vi "Sensor Setting.vi"(8 "error in":errorcluster) -> (0 "error  out":errorcluster)   [LabVIEW 2015]
uses:
  Control Button/Save.ctl
  Control Button/Exit.ctl
  <vilib>/addons/database/Connection.llb/DB Tools Open Connec (String).vi
  Galobal variable_TI.vi
  <vilib>/addons/database/_DB Variant To Data/Database Variant To Data.xnode
  <vilib>/addons/database/NI_Database_API.lvlib
panel:
  out "error out":errorcluster
  in  "Model":string(combo)
  in  "Setting Data":T1
  in  "String":string
  in  "Cluster 3":T1
  out "Model":string
  in  "Exit":T2
  in  "Save":T3
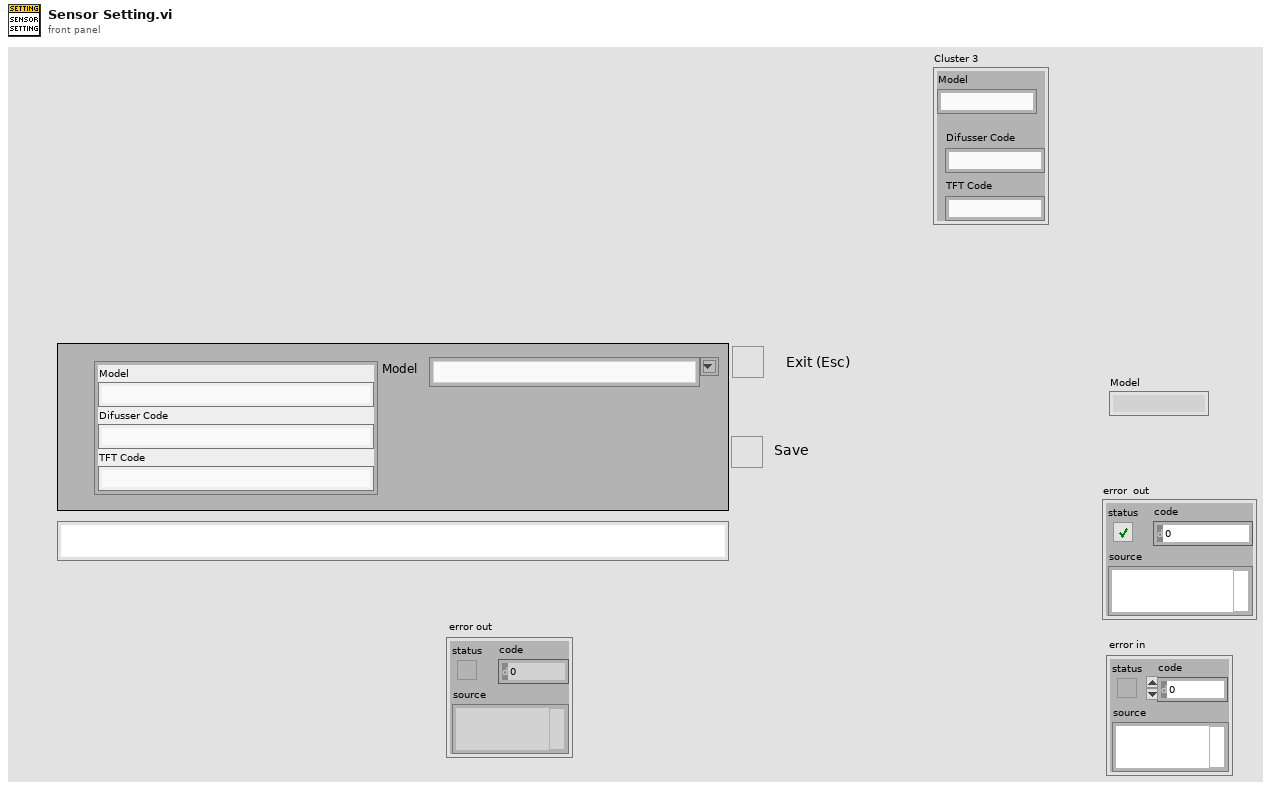
[diagram p1: front panel]
types:
  T1 = cluster{"Model":string, "Difusser Code":string, "TFT Code ":string}
  T2 = typedef "Exit.ctl" = bool
  T3 = typedef "Save.ctl" = bool
  T4 = typedef "NI_Database_API.lvlib/Conn ObjectReference.ctl" = refnum<k1>
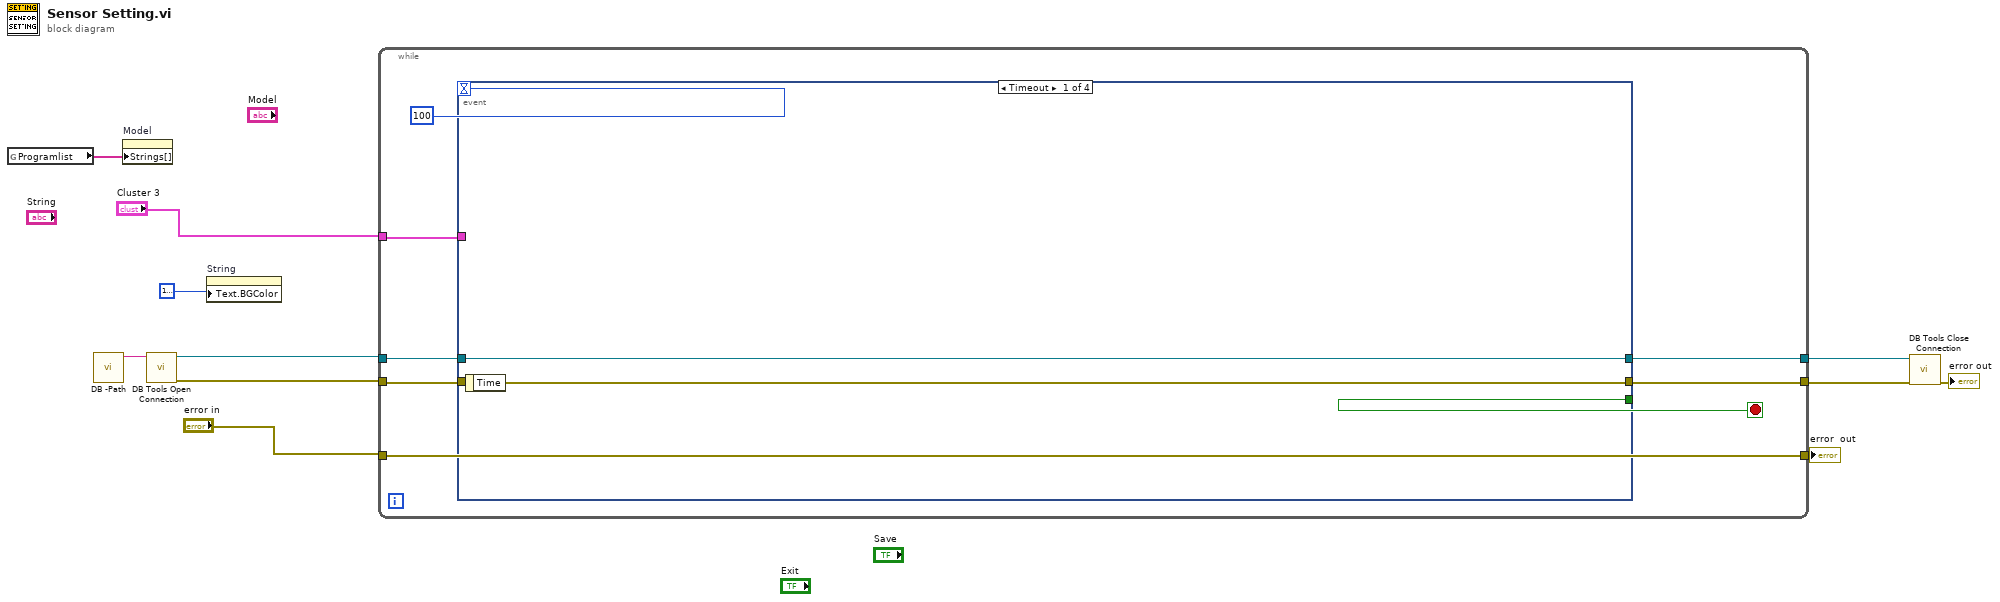
[diagram p0: block diagram]
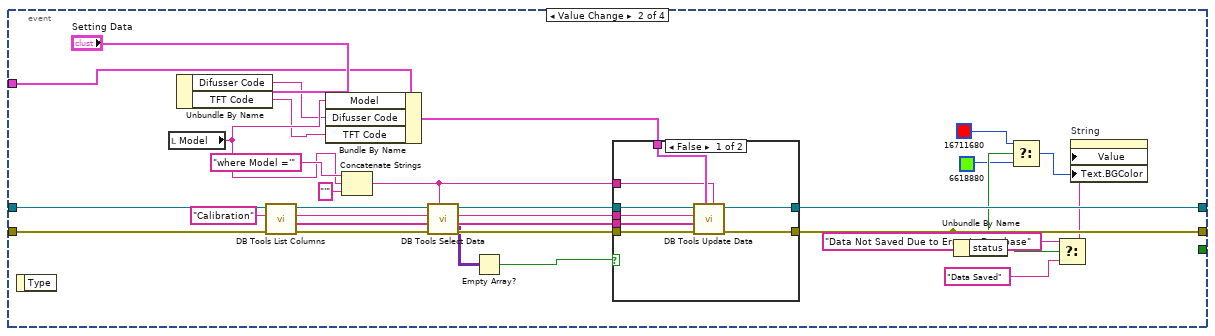
[diagram p2: hidden frame]
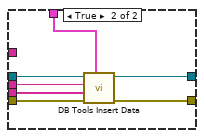
[diagram p3: hidden frame]
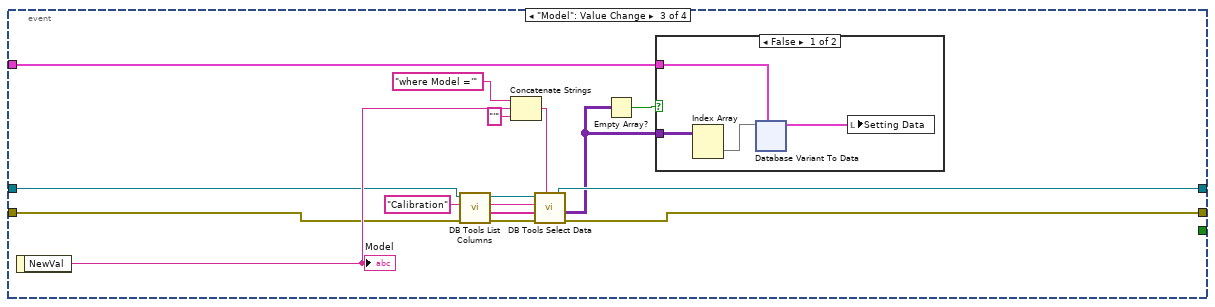
[diagram p4: hidden frame]
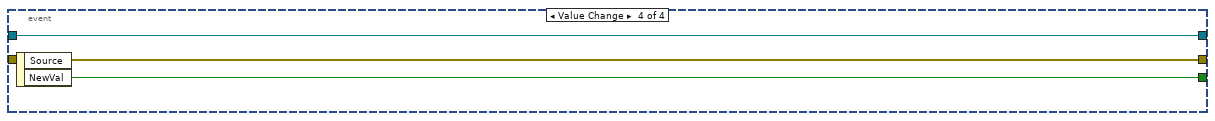
[diagram p6: hidden frame]
diagram:
  n1 = global read "Galobal variable_TI.vi" "Programlist"() -> (w6:string[])
  n2 = call "DB -Path.vi"() -> ("String"=w11:string)  [unwired: 11 in]
  n3 = property on="Model" class="CmbBox"("Strings[]"=w6) -> ()  [unwired: 2 in, 2 out]
  n4 = call-poly <vilib>:"DB Tools Open Connection.vi"("connection information"=w11) -> ("error out"=w9:errorcluster, "connection reference"=w10:T4)  [unwired: 7 in]
  n5 = property on="String" class="Str"("Text.BGColor"=u32 16777226 ("Color Box")) -> ()  [unwired: 2 in, 2 out]
  n6 = while {
    tunnel: w10 -> [w18]
    tunnel: w9 -> [w17]
    tunnel: [w16] -> w8
    tunnel: [w15] -> w7
    tunnel: "error in" -> [w13]
    tunnel: [w13] -> w4
    tunnel: "Cluster 3" -> [w12]
    stop <- w14 stop-if-true
    n7 = event shown="[0] Timeout" {
      selector: _ -> [_ _ _ _]
      dyn-events: _ -> [_ _ _ _]
      timeout: 100 -> [_ _ _ _]
      tunnel: w18 -> [w21 w49 w71 w182]
      tunnel: w17 -> [w20 w48 w70 w183]
      tunnel: [w21 w47 w69 w182] -> w16
      tunnel: [w20 w38 w68 w183] -> w15
      tunnel: [_ _ _ w181] -> w14
      tunnel: w12 -> [_ w41 w67 _]
      event Timeout {
        n8 = event-data() -> ()  [unwired: 1 in, 1 out]
      }
      event Value Change {
        w25 = "Calibration" ("table")
        n9 = event-data() -> ()  [unwired: 1 in, 1 out]
        n10 = local read "Model"() -> (w42:string)
        n11 = Unbundle By Name("Setting Data") -> ("Difusser Code"=w40:string, "TFT Code"=w39:string)
        n12 = call <vilib>:"DB Tools List Columns.vi"("error in (no error)"=w48, "table"=w25, "connection reference"=w49) -> ("error out"=w28:errorcluster, "columns"=w29:string[], "connection reference out"=w30:T4)  [unwired: 1 in, 1 out]
        n13 = Bundle By Name(cluster=w41, "Model"=w42, "Difusser Code"=w40, "TFT Code"=w39) -> (w45:T1)
        n14 = Concatenate Strings("where Model ='" ("string"), w42, "'" ("string")) -> (w24:string)
        n15 = call <vilib>:"DB Tools Select Data.vi"("condition"=w24, "error in (no error)"=w28, "columns"=w29, "table"=w25, "connection reference"=w30) -> ("error out"=w27:errorcluster, "data"=w23:variant[][], "connection reference out"=w26:T4)  [unwired: 1 in]
        n16 = Empty Array?(array=w23) -> (empty?=w22:bool)
        n17 = case shown="False" w22 {
          tunnel: [w57 w60] -> w47
          tunnel: w45 -> [w56 w58]
          tunnel: [w55 w59] -> w38
          tunnel: w29 -> [w54 w61]
          tunnel: w27 -> [w53 w63]
          tunnel: w26 -> [w52 w64]
          tunnel: w25 -> [w51 w62]
          tunnel: w24 -> [w50 _]
          frame False {
            n18 = call <vilib>:"DB Tools Update Data.vi"("condition"=w50, "data"=w56, "error in (no error)"=w53, "columns"=w54, "table"=w51, "connection reference"=w52) -> ("error out"=w55:errorcluster, "connection reference out"=w57:T4)  [unwired: 4 in]
          }
          frame True {
            n19 = call <vilib>:"DB Tools Insert Data.vi"("data"=w58, "error in (no error)"=w63, "columns"=w61, "table"=w62, "connection reference"=w64) -> ("error out"=w59:errorcluster, "connection reference out"=w60:T4)  [unwired: 5 in]
          }
        }
        n20 = Unbundle By Name(w38) -> ("status"=w34:bool)
        n21 = Select(t=u32 16711680 ("Color Box"), s=w34, f=u32 6618880 ("Color Box")) -> (s? t:f=w31:u32)
        n22 = Select(t="Data Not Saved Due to Error In Database", s=w34, f="Data Saved") -> (s? t:f=w35:string)
        n23 = property on="String" class="Str"("Value"=w35, "Text.BGColor"=w31) -> ()  [unwired: 2 in, 2 out]
      }
      event "Model": Value Change {
        w73 = "Calibration" ("table")
        n24 = event-data() -> ("NewVal"=w72:string)  [unwired: 1 in]
        "Model" <- w72
        n25 = call <vilib>:"DB Tools List Columns.vi"("error in (no error)"=w70, "table"=w73, "connection reference"=w71) -> ("error out"=w79:errorcluster, "columns"=w77:string[], "connection reference out"=w78:T4)  [unwired: 1 in, 1 out]
        n26 = Concatenate Strings("where Model ='" ("string"), w72, "'" ("string")) -> (w74:string)
        n27 = call <vilib>:"DB Tools Select Data.vi"("condition"=w74, "error in (no error)"=w79, "columns"=w77, "table"=w73, "connection reference"=w78) -> ("error out"=w68:errorcluster, "data"=w66:variant[][], "connection reference out"=w69:T4)  [unwired: 1 in]
        n28 = Empty Array?(array=w66) -> (empty?=w65:bool)
        n29 = case shown="False" w65 {
          tunnel: w66 -> [w83 _]
          tunnel: w67 -> [w81 _]
          frame False {
            n30 = Index Array(array=w83) -> (element=w82:variant[])  [unwired: 2 in]
            n31 = xnode "Database Variant To Data"("database variant"=w82, "type"=w81) -> ("data"=w80:T1)  [unwired: 1 in, 1 out]
            n32 = local write "Setting Data"(w80) -> ()
          }
          frame True {
          }
        }
      }
      event Value Change {
        n33 = event-data() -> ("NewVal"=w181:T2)  [unwired: 1 in, 1 out]
      }
    }
  }
  "error  out" <- w4
  n34 = call <vilib>:"DB Tools Close Connection.vi"("error in (no error)"=w7, "connection reference"=w8) -> ("error out"=→"error out":errorcluster)  [unwired: 5 in]
